vi "whileloopStructureExample2.vi"() -> ()   [LabVIEW 2014]
panel:
  out "Output Array\nIndicator":dbl[](array[numeric])
  in  "Stop Value\nControl":dbl
  in  "Start Value\nControl":dbl
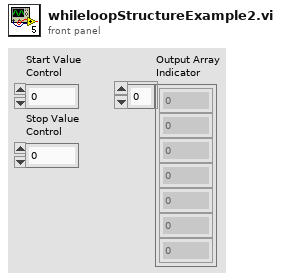
[diagram p1: front panel]
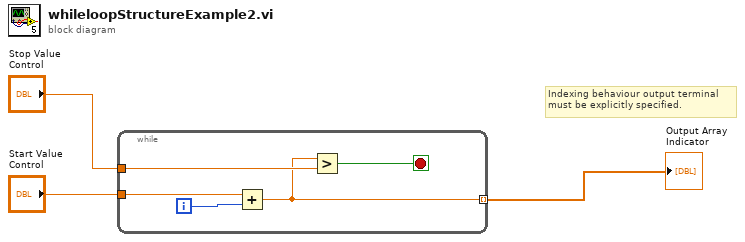
[diagram p0: block diagram]
diagram:
  # "Indexing behaviour output terminal\nmust be explicitly specified."
  n1 = while {
    tunnel: "Start Value\nControl" -> [w8]
    tunnel: "Stop Value\nControl" -> [w5]
    tunnel: [w4] -> w1 mode=indexing
    i -> [w7]
    stop <- w6 stop-if-true
    n2 = Add(x=w8, y=w7) -> (x+y=w4:dbl)
    n3 = Greater?(x=w4, y=w5) -> (0:w6:bool)
  }
  "Output Array\nIndicator" <- w1
